vi "GetLoadModelMode.vi"(8 "error in (no error)":errorcluster, 11 "GenericController in":refnum<class "GenericController.lvclass">) -> (0 "error out":errorcluster, 2 "LoadDemoModel":bool, 3 "GenericController out":refnum<class "GenericController.lvclass">)   [LabVIEW 2020, in "GenericController.lvlib" / "GenericController.lvclass"]
uses:
  GenericController.lvclass
  GenericController.lvclass/GenericController.ctl
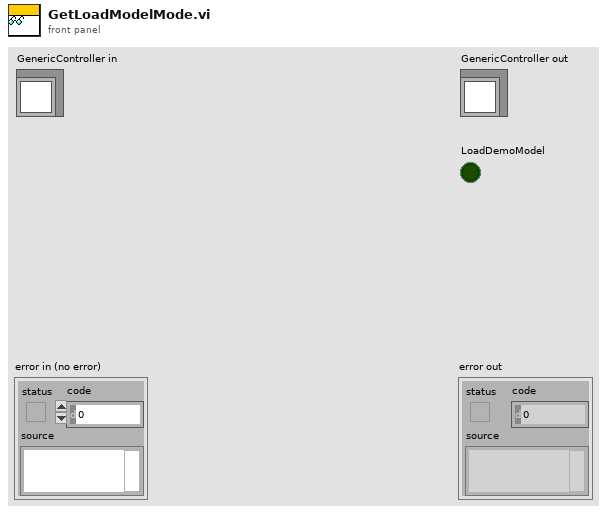
[diagram p1: front panel]
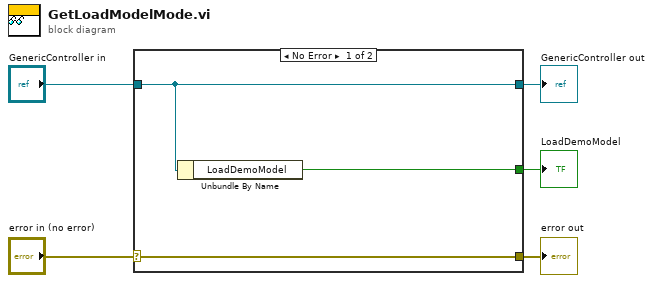
[diagram p0: block diagram]
diagram:
  n1 = case shown="No Error" "error in (no error)" {
    selector: "error in (no error)" -> [w8 w9]
    tunnel: [w8 w9] -> w4
    tunnel: [w7 w10] -> w2
    tunnel: "GenericController in" -> [w7 w10]
    tunnel: [w6 _] -> w1
    frame No Error {
      n2 = Unbundle By Name(w7) -> ("LoadDemoModel"=w6:bool)
    }
    frame Error {
    }
  }
  "error out" <- w4
  "GenericController out" <- w2
  "LoadDemoModel" <- w1
